vi "Multi_OUI_NON.vi"(8 "errin":errorcluster caption="entrée d'erreur (pas d'erreur)", 9 "errinb":bool, 10 "Tableau":string[](array[string])) -> (0 "errout":errorcluster caption="sortie d'erreur", 3 "isok?":bool)   [LabVIEW 2020]
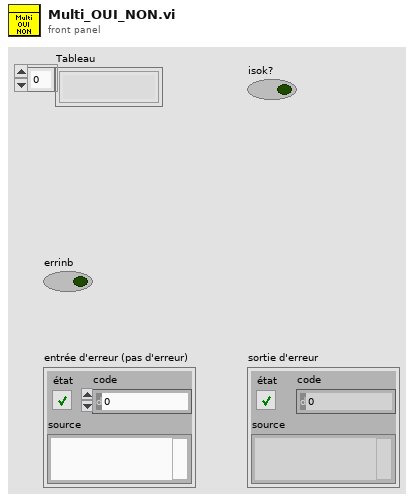
[diagram p1: front panel]
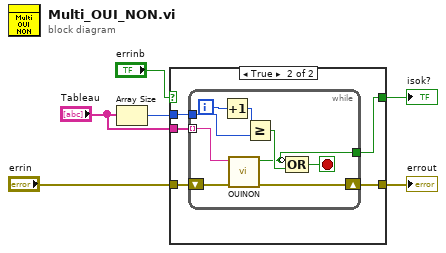
[diagram p0: block diagram]
diagram:
  n1 = Array Size(array="Tableau") -> (size(s)=w1:i32)
  n2 = case shown="True" "errinb" {
    selector: "errinb" -> [w7 _]
    tunnel: "Tableau" -> [_ w13]
    tunnel: w1 -> [_ w12]
    tunnel: [w7 w11] -> w3
    tunnel: [w8 w10] -> w4
    tunnel: "errin" -> [w8 w9]
    frame False {
    }
    frame True {
      n3 = while {
        tunnel: w13 -> [w20] mode=indexing
        tunnel: w12 -> [w21]
        shift-right: [w18] -> w10
        shift-left: w9 -> [w19]
        tunnel: [w15] -> w11
        i -> [w22]
        stop <- w16 stop-if-true
        n4 = Increment(x=w22) -> (x+1=w14:i32)
        n5 = call <userlib>:"OUINON.vi"("errin"=w19, "image"=w20) -> ("error out"=w18:errorcluster, "OUI/NON"=w15:bool)  [unwired: 8 in]
        n6 = Greater Or Equal?(x=w14, y=w21) -> (x >= y?=w17:bool)
        n7 = Compound Arithmetic op=OR ("Opérateur arithmétique")(invert w15, w17) -> (w16:bool)
      }
    }
  }
  "errout" <- w4
  "isok?" <- w3
